vi "LabVIEWRTControlStartupVI.vi"() -> ()   [LabVIEW 2014]
doc: "This example demonstrates a command based communication architecture using TCP. It shows a protocol for packaging and parsing data while minimizing network traffic. Refer to the National Instruments Web site at ni.com/info and enter the info code \"commtcp\" for more information about this command based communication architecture."
uses:
  Control 2.ctl
  ChannelCommand.ctl
  Control 1.ctl
  WaveType.ctl
  MoterEnable.ctl
  <userlib>/VMIC/VMIC 5565 Reflective Memory.llb/VMIC Reference.ctl
  <vilib>/Platform/TimedLoop/XDataNode/timing_clust.ctl
  <vilib>/Platform/TimedLoop/XDataNode/nitl_modes.ctl
  <vilib>/Platform/TimedLoop/XDataNode/wakeup.ctl
  <vilib>/DAQmx/write.llb/DAQmx Write (Analog 1D DBL NChan 1Samp).vi
  <userlib>/VMIC/VMIC 5565 Reflective Memory.llb/VMIC Write (U32).vi
  <vilib>/DAQmx/write.llb/DAQmx Write (Digital 1D Bool NChan 1Samp 1Line).vi
  <userlib>/VMIC/VMIC 5565 Reflective Memory.llb/VMIC Read (U8).vi
  <vilib>/Platform/TimedLoop/XDataNode/XDataNode.xnode
  <vilib>/Platform/TimedLoop/XDataNode/XDNodeRunTimeDep.lvlib
  <vilib>/real-time/NI_Real-Time Libraries.lvlib
  <vilib>/NI_Real-Time Target Support.lvlib
  <vilib>/real-time/rtutility.llb/RT Restart Target (Self).vi
panel:
  out "Protect":bool
  out "x = y?":bool
  out "error out 12":errorcluster caption="错误输出"
  out "number of samples written per channel":u32
  out "error out 11":errorcluster caption="error out"
  out "error out 10":errorcluster caption="error out"
  out "error out 9":errorcluster caption="error out"
  out "上传数组":dbl[](array[numeric])
  out "VMIC write":sgl[](array[numeric])
  out "6612counterTask 8":refnum<k21>
  out "6612counterTask 7":refnum<k21>
  out "6612counterTask 6":refnum<k21>
  out "6612counterTask 5":refnum<k21>
  out "ResetAforce":dbl[](array[numeric])
  out "x/y":dbl
  out "全局结束时间":i64
  out "实际结束[i-1]":i64
  out "延迟完成？[i-1]":bool
  out "超时":i32=-1
  out "6612counterTask 4":refnum<k21>
  out "6612counterTask 3":refnum<k21>
  out "6612counterTask 2":refnum<k21> caption="任务输出"
  out "6612counterTask":refnum<k21>
  out "x与y? 4":bool[](array[boolean])
  out "x与y? 3":bool[](array[boolean])
  out "VMIC reference":T1
  out "PXI6363IO":refnum<k21>
  out "x与y?":bool[](array[boolean])
  out "error out 6":errorcluster caption="error out"
  out "error out 4":errorcluster
  out "OutPut":dbl[](array[numeric])
  out "Command Type":i32
  out "Msg Head":string
  out "error out":errorcluster caption="错误输出"
  out "长度 3":i32
  out "长度 2":i32
  out "长度":i32
  out "connection ID":refnum<k5> caption="连接ID"
  out "6363Task":refnum<k21> caption="任务输出"
  out "error out 3":errorcluster caption="错误输出"
  out "加速度信号":dbl[](array[numeric])
  out "同步信号":dbl[](array[numeric])
  out "轴向位移":dbl[](array[numeric])
  out "轴向力":dbl[](array[numeric])
  out "T_outrange":bool[](array[boolean])
  out "error out 8":errorcluster caption="error out"
  out "error out 7":errorcluster caption="error out"
  out "error out 5":errorcluster caption="错误输出"
  out "diff syn out 2":dbl[](array[numeric])
  out "Forward":dbl[](array[numeric])
  out "AngleSampleData 2":dbl[](array[numeric])
  out "TorqueSampledata 2":dbl[](array[numeric])
  out "control out":dbl[](array[numeric])
  out "command out 2":dbl[](array[numeric])
  out "Wave out 2":dbl[](array[numeric])
  out "type out":dbl[](array[numeric])
  out "Enable":bool[](array[boolean])
  out "syn out":dbl[](array[numeric])
  out "TempAnOut":dbl[](array[numeric])
  out "StartChannelReset":bool[](array[boolean])
  out "retorquedata2":dbl[](array[numeric])
  out "reangeldata2":dbl[](array[numeric])
  out "output 4":dbl[](array[numeric])
  out "TestLoops 2":i32
  out "ResetAngle":dbl[](array[numeric])
  out "ResetTorque":dbl[](array[numeric])
  out "error out 2":errorcluster
  in  "Exit":bool
  out "ControlPara":dbl[][](array[numeric])
  out "ChannelSetArray":T2 {"Enable" items=["不使能", "使能"]; "Wave" items=["0指令", "正弦波", "方波", "三角波", "常值", "波形数据", "白噪声", "正弦扫频", "梯度加载", "VMIC"]; "ChannelType" items=["标准波形跟踪"=1, "扫频测试"=2, "消除多余力"=3, "梯度加载"=4, "载荷谱跟踪"=5, "模拟输入跟踪"=9]; "ChannelStatus" items=["通道关", "位置通道", "加载通道"]}
  out "Stop":bool
  out "iCommand":i32
  out "TestLoops":i32
  out "dt":dbl
  out "PXI6733Task":refnum<k21>
  out "Data array":dbl[][](array[numeric])
  out "error  out":errorcluster
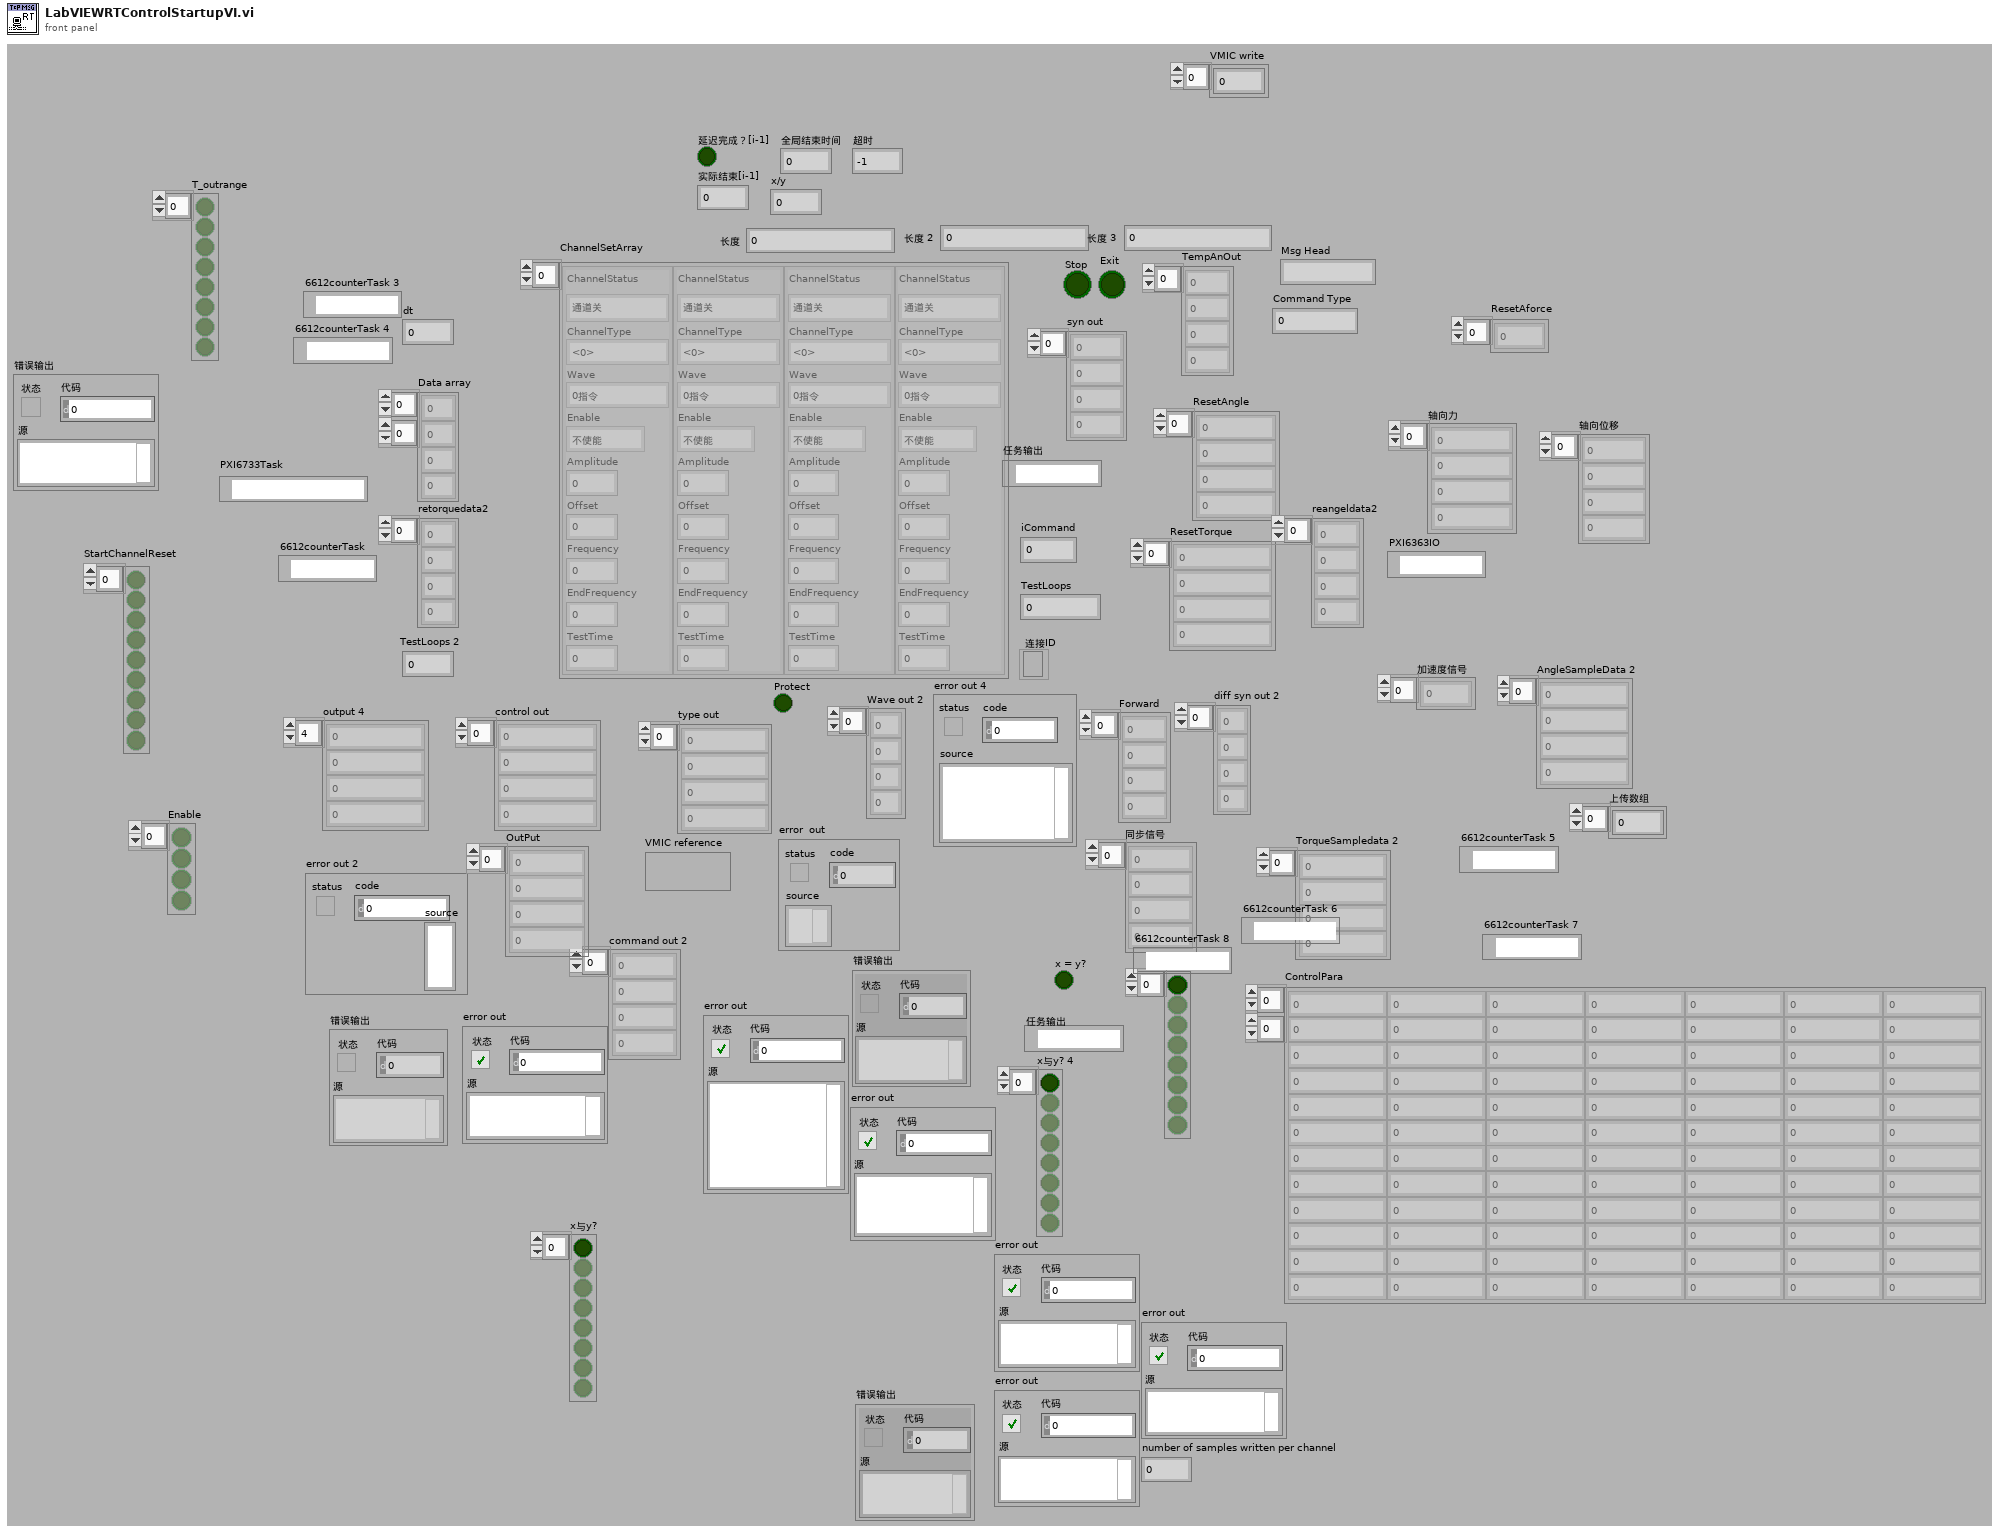
[diagram p1: front panel]
types:
  T1 = typedef "VMIC Reference.ctl" = variant
  T2 = typedef "Control 2.ctl" = T3[]
  T3 = typedef "ChannelCommand.ctl" = cluster{"ChannelStatus":T4, "ChannelType":i32, "Wave":T5, "Enable":T6, "Amplitude":dbl, "Offset":dbl, "Frequency":dbl, "EndFrequency":dbl, "TestTime":dbl}
  T4 = typedef "Control 1.ctl" = i32
  T5 = typedef "WaveType.ctl" = i32
  T6 = typedef "MoterEnable.ctl" = u16
  T7 = typedef "XDNodeRunTimeDep.lvlib/timing_clust.ctl" = cluster{"Expected End [f-1]":u64, "Actual End [f-1]":u64, "Finished Late? [f-1]":bool, "Expected End [i-1]":u64, "Actual End [i-1]":u64, "Finished Late? [i-1]":bool, "Expected Start [i]":u64, "Actual Start [i]":u64, "Expected Start [f]":u64, "Actual Start [f]":u64, "Source Name":string, "Structure Name":string, "Period":i64, "Deadline":i64, "Offset":i64, "Start":i64, "Priority":i32, "Timeout":i32, "Mode":T8, "Wakeup Reason":T9, "Error":errorcluster, "Source Type":string, "Secondary Source Type":string, "Global End Time":u64, "Global Start Time":u64, "Frame Duration":u64, "Iteration Duration":u64, "Assigned CPU":i32, "I/O Scan Engine Mode":u32}
  T8 = typedef "XDNodeRunTimeDep.lvlib/nitl_modes.ctl" = enum32{"No Change", "Process missed periods, maintain original phase", "Discard missed periods, maintain original phase", "Process missed periods, ignore original phase", "Discard missed periods, ignore original phase"}
  T9 = typedef "XDNodeRunTimeDep.lvlib/wakeup.ctl" = enum32{"Normal", "Aborted", "Asynchronous wakeup", "Timing source error", "Timed loop error", "Timeout"}
  T10 = enum16{"big-endian, network order", "native, host order", "little-endian"}
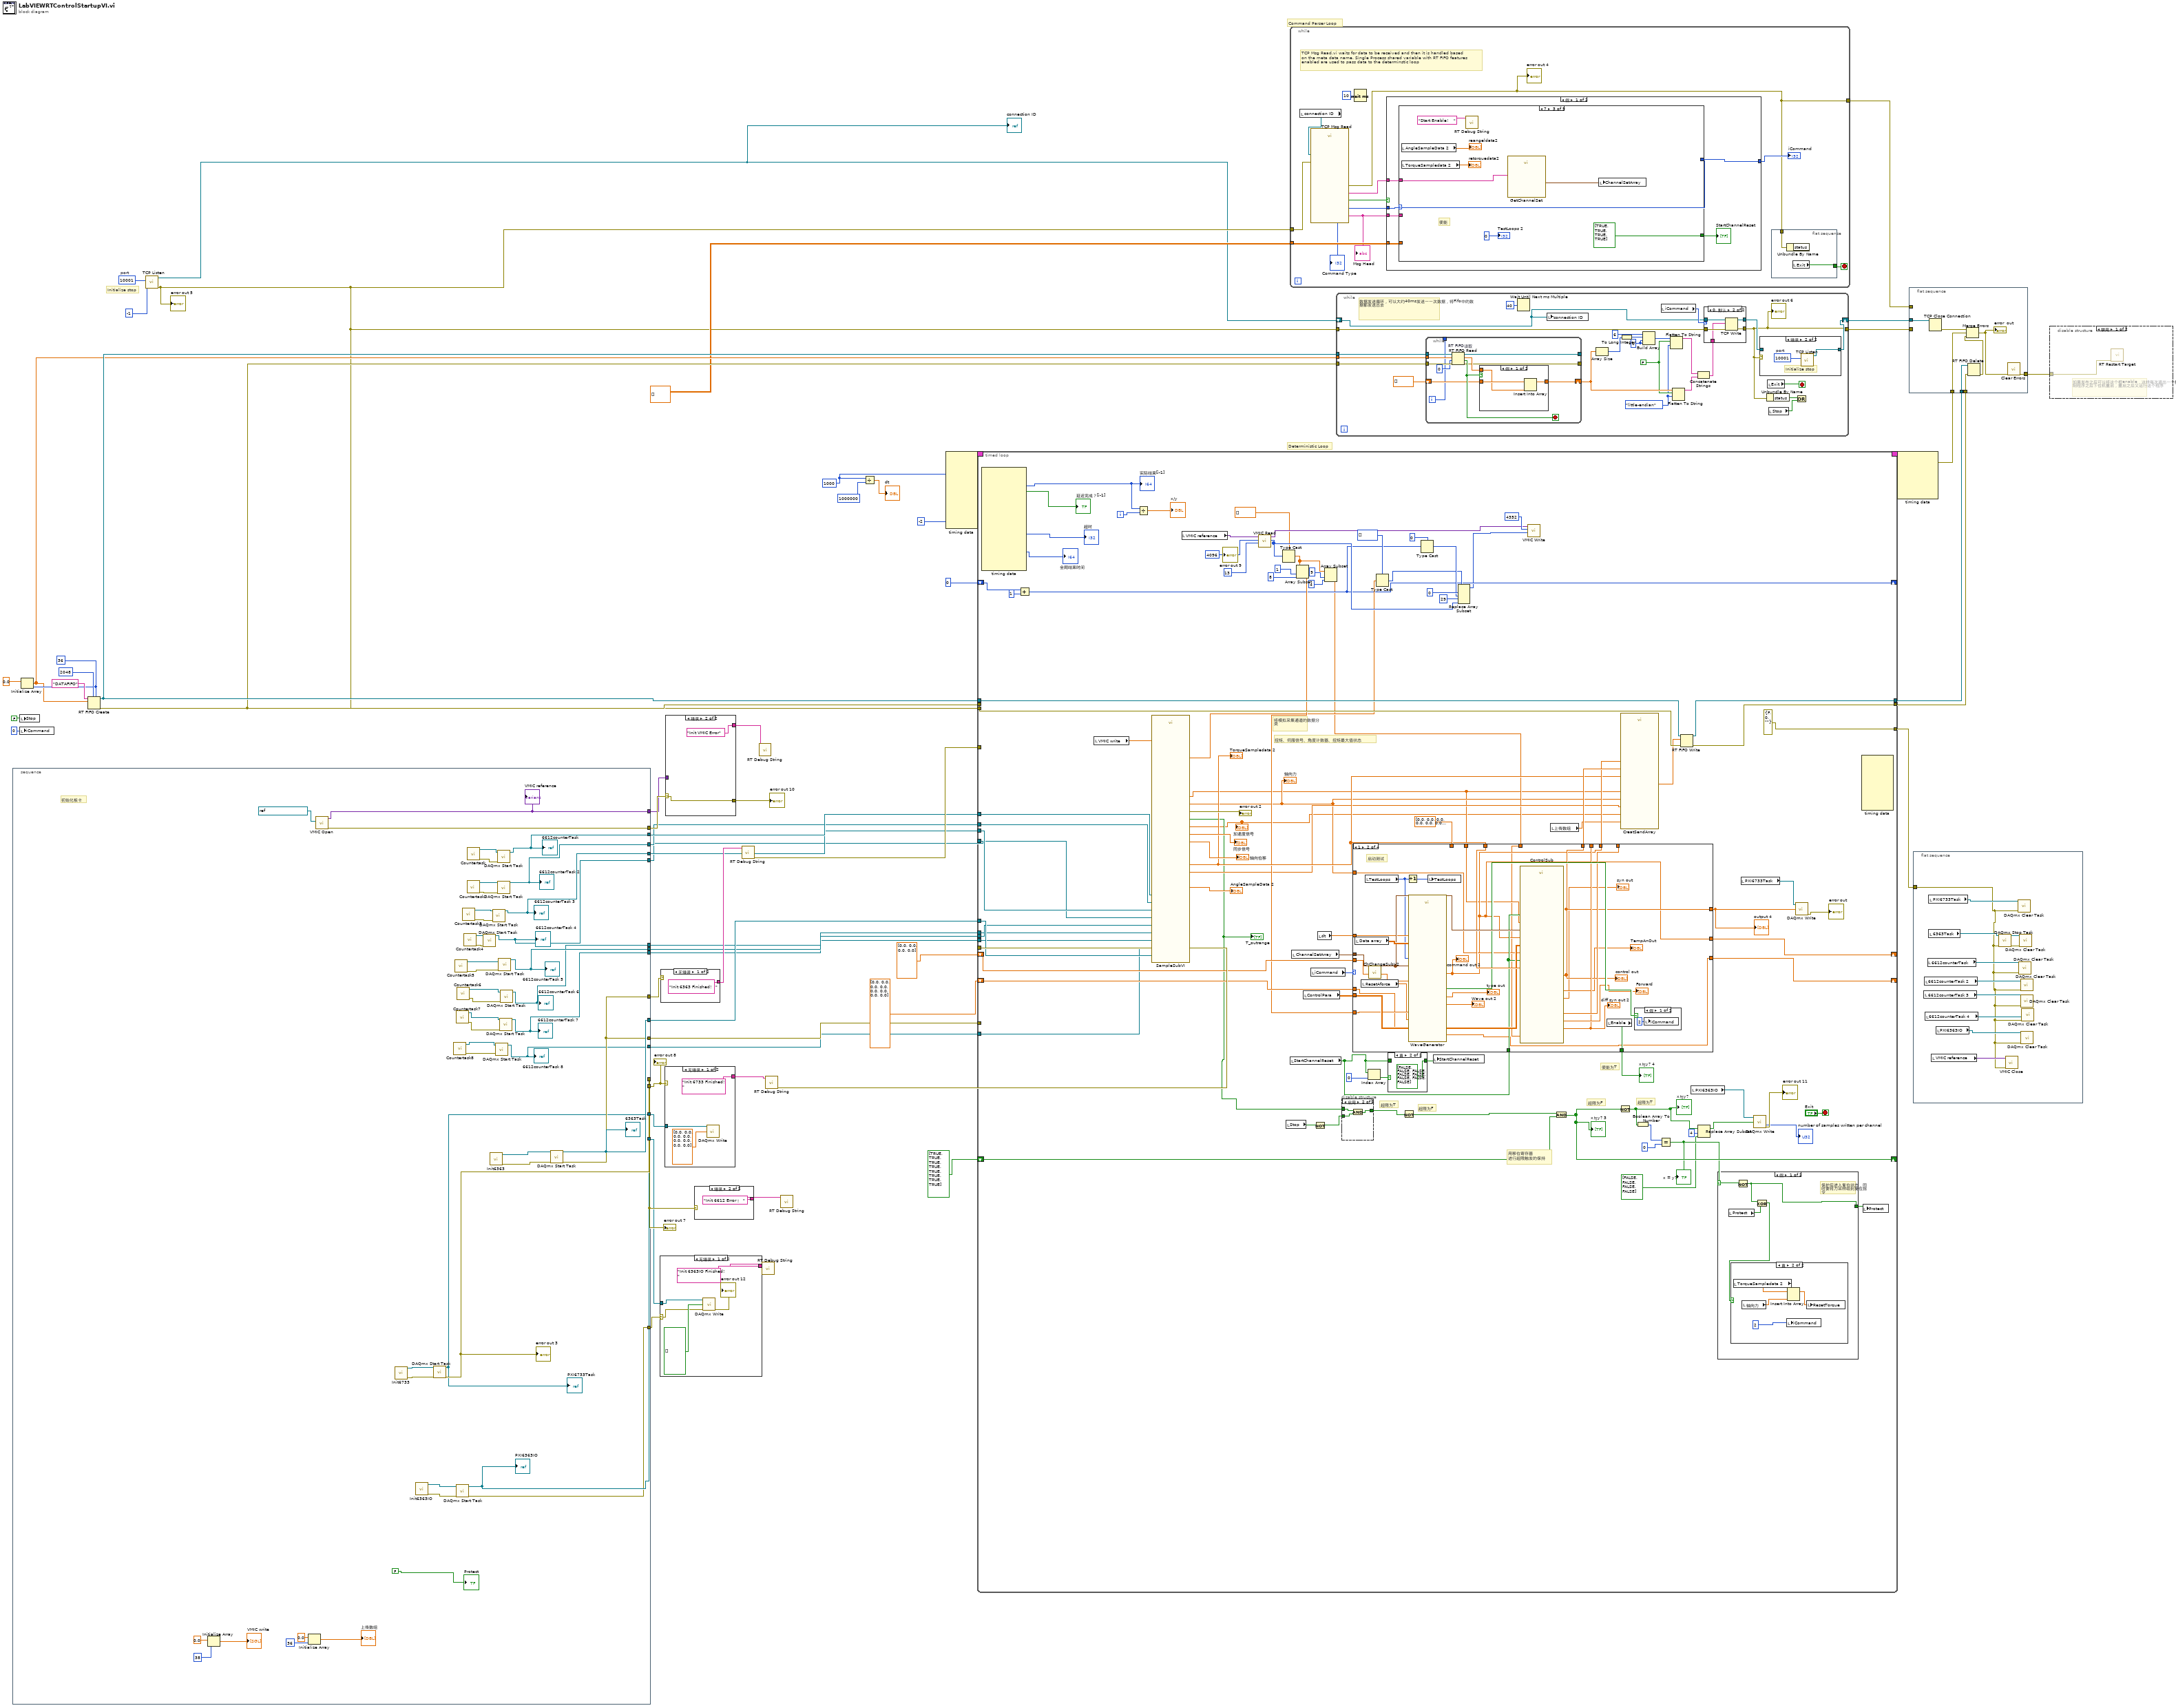
[diagram p0: block diagram]
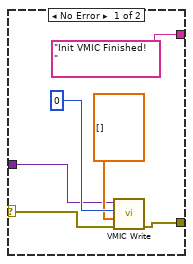
[diagram p2: hidden frame]
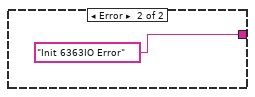
[diagram p3: hidden frame]
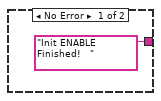
[diagram p4: hidden frame]
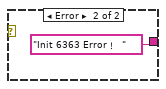
[diagram p5: hidden frame]
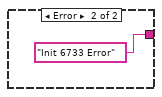
[diagram p7: hidden frame]
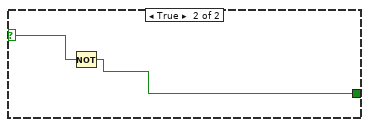
[diagram p9: hidden frame]
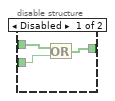
[diagram p10: hidden frame]
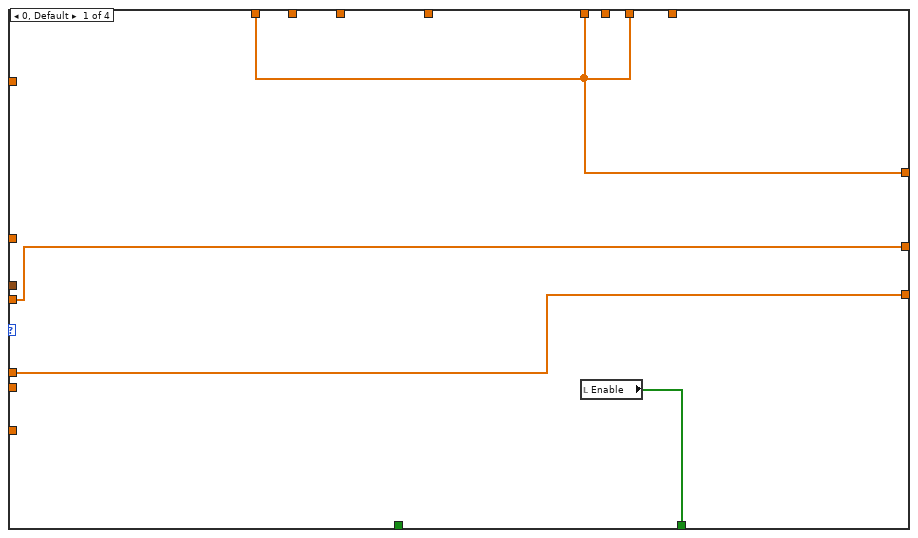
[diagram p12: hidden frame]
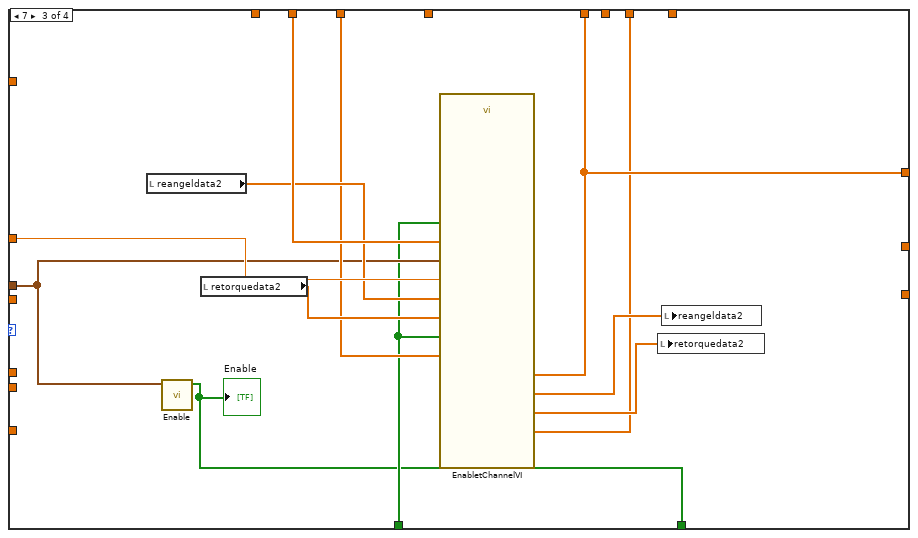
[diagram p14: hidden frame]
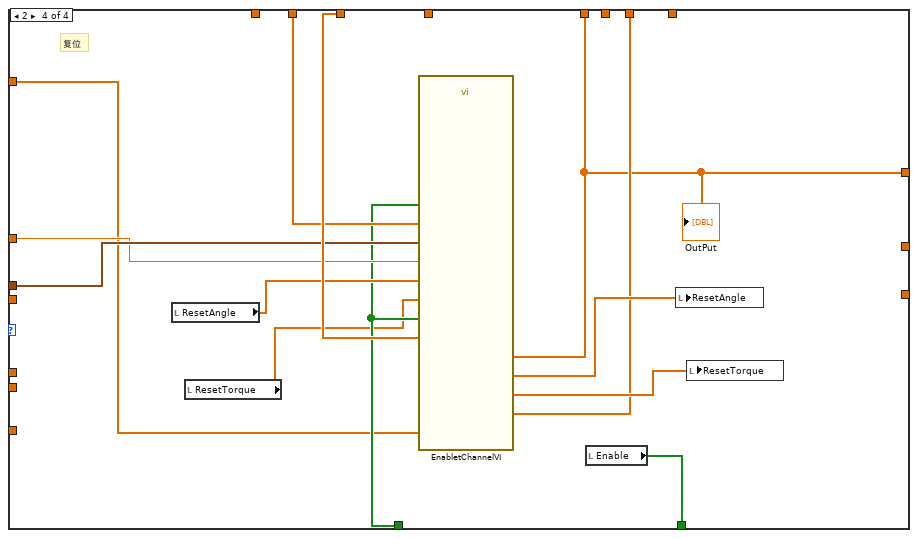
[diagram p15: hidden frame]
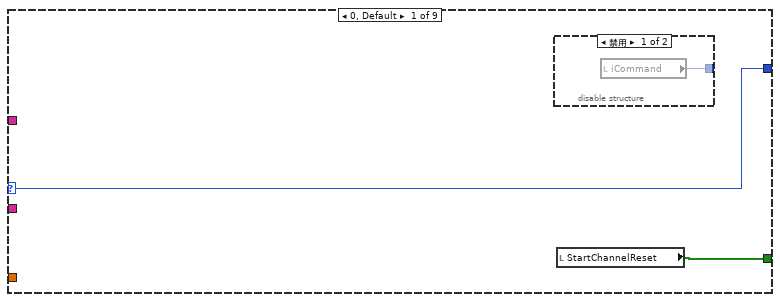
[diagram p16: hidden frame]
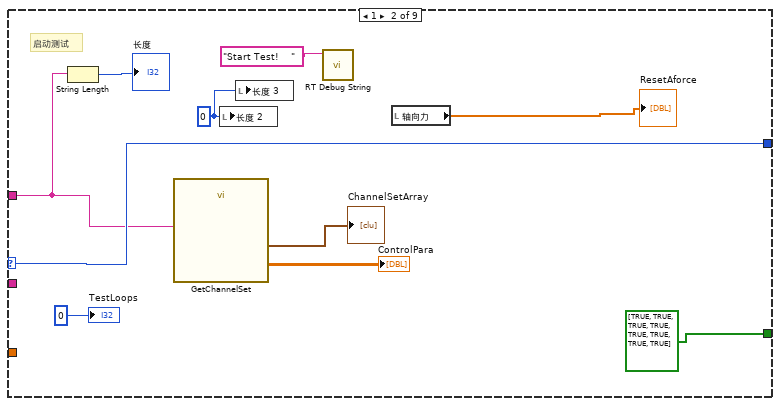
[diagram p18: hidden frame]
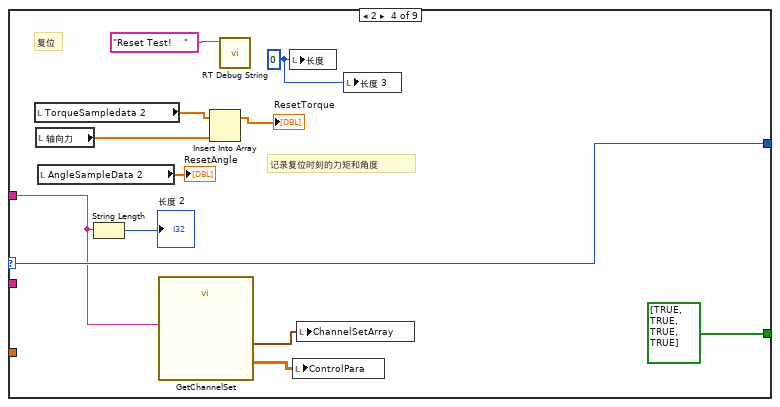
[diagram p19: hidden frame]
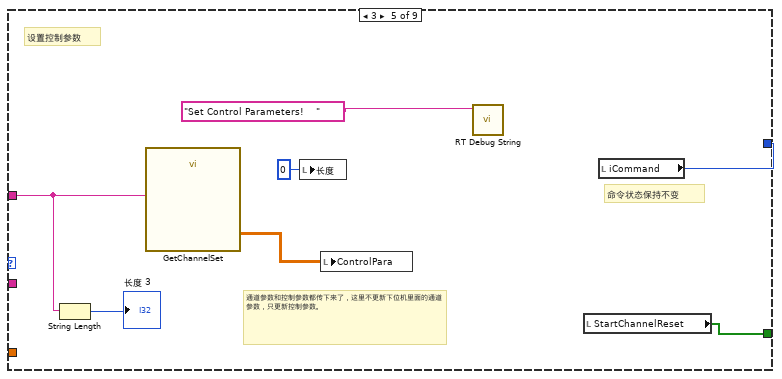
[diagram p20: hidden frame]
diagram:
  w46 = u32 36 ("elements in array (1)")
  w54 = i64 1000 ("Period")
  w58 = u16 10001  # port
  # "Deterministic Loop"
  # "Initialize stop"
  # "Command Parser Loop"
  n1 = stacked-sequence {
    tunnel: [w87] -> w25
    tunnel: [w87] -> w28
    tunnel: [w88] -> w24
    tunnel: [w85] -> w23
    tunnel: [w88] -> w9
    tunnel: [w89] -> w22
    tunnel: [w81] -> w17
    tunnel: [w83] -> w19
    tunnel: [w103] -> w16
    tunnel: [w102] -> w15
    tunnel: [w93] -> w13
    tunnel: [w92] -> w12
    tunnel: [w91] -> w11
    tunnel: [w90] -> w10
    tunnel: [w69] -> w8
    tunnel: [w68] -> w7
    tunnel: [w67] -> w6
    tunnel: [w66] -> w5
    frame #0 {
      # "初始化板卡"
      n2 = Initialize Array(sgl 0.0 ("元素"), 38 ("维数大小")) -> (→"VMIC write":sgl[])
      n3 = Initialize Array(0.0 ("element"), 36 ("dimension size")) -> (→"上传数组":dbl[])
      n4 = call <userlib>:"VMIC Open.vi"("VISA resource name (empty)"=refnum<visa-resource-name> "PXI13::12::INSTR") -> ("error out"=w103:errorcluster, "VMIC reference"=w102:T1)  [unwired: 5 in]
      "VMIC reference" <- w102
      n5 = call "Init6733.vi"() -> ("error out"=w84:errorcluster, "task out"=w86:refnum<k21>)  [unwired: 10 in]
      n6 = call "Init6363IO.vi"() -> ("error out"=w80:errorcluster, "task out"=w82:refnum<k21>)  [unwired: 10 in]
      n7 = call <vilib>:"DAQmx Start Task.vi"("task/channels in"=w86, "error in"=w84) -> ("task out"=w85:refnum<k21>, "error out"=w87:errorcluster)  [unwired: 12 in]
      "PXI6733Task" <- w85
      "error out 3" <- w87
      n8 = call "Countertask8.vi"() -> ("error out"=w70:errorcluster, "task out"=w71:refnum<k21>)  [unwired: 10 in]
      n9 = call "Countertask5.vi"() -> ("error out"=w76:errorcluster, "task out"=w77:refnum<k21>)  [unwired: 10 in]
      n10 = call "Countertask7.vi"() -> ("error out"=w72:errorcluster, "task out"=w73:refnum<k21>)  [unwired: 10 in]
      n11 = call <vilib>:"DAQmx Start Task.vi"("task/channels in"=w82, "error in"=w80) -> ("task out"=w83:refnum<k21>, "error out"=w81:errorcluster)  [unwired: 12 in]
      "PXI6363IO" <- w83
      n12 = call "Countertask6.vi"() -> ("error out"=w74:errorcluster, "task out"=w75:refnum<k21>)  [unwired: 10 in]
      n13 = call "Countertask3.vi"() -> ("error out"=w96:errorcluster, "task out"=w97:refnum<k21>)  [unwired: 10 in]
      n14 = call "Countertask4.vi"() -> ("error out"=w94:errorcluster, "task out"=w95:refnum<k21>)  [unwired: 10 in]
      n15 = call "Countertask2.vi"() -> ("error out"=w98:errorcluster, "task out"=w99:refnum<k21>)  [unwired: 10 in]
      n16 = call "Countertask.vi"() -> ("error out"=w100:errorcluster, "task out"=w101:refnum<k21>)  [unwired: 10 in]
      n17 = call <vilib>:"DAQmx Start Task.vi"("task/channels in"=w95, "error in"=w94) -> ("task out"=w90:refnum<k21>)  [unwired: 12 in, 1 out]
      "6612counterTask 4" <- w90
      n18 = call "Init6363.vi"() -> ("error out"=w78:errorcluster, "task out"=w79:refnum<k21>)  [unwired: 10 in]
      n19 = call <vilib>:"DAQmx Start Task.vi"("task/channels in"=w97, "error in"=w96) -> ("task out"=w91:refnum<k21>)  [unwired: 12 in, 1 out]
      "6612counterTask 3" <- w91
      n20 = call <vilib>:"DAQmx Start Task.vi"("task/channels in"=w71, "error in"=w70) -> ("task out"=w66:refnum<k21>)  [unwired: 12 in, 1 out]
      "6612counterTask 8" <- w66
      n21 = call <vilib>:"DAQmx Start Task.vi"("task/channels in"=w101, "error in"=w100) -> ("task out"=w93:refnum<k21>)  [unwired: 12 in, 1 out]
      "6612counterTask" <- w93
      n22 = call <vilib>:"DAQmx Start Task.vi"("task/channels in"=w99, "error in"=w98) -> ("task out"=w92:refnum<k21>)  [unwired: 12 in, 1 out]
      "6612counterTask 2" <- w92
      n23 = call <vilib>:"DAQmx Start Task.vi"("task/channels in"=w77, "error in"=w76) -> ("task out"=w69:refnum<k21>)  [unwired: 12 in, 1 out]
      "6612counterTask 5" <- w69
      n24 = call <vilib>:"DAQmx Start Task.vi"("task/channels in"=w73, "error in"=w72) -> ("task out"=w67:refnum<k21>)  [unwired: 12 in, 1 out]
      "6612counterTask 7" <- w67
      n25 = call <vilib>:"DAQmx Start Task.vi"("task/channels in"=w75, "error in"=w74) -> ("task out"=w68:refnum<k21>)  [unwired: 12 in, 1 out]
      "6612counterTask 6" <- w68
      n26 = call <vilib>:"DAQmx Start Task.vi"("task/channels in"=w79, "error in"=w78) -> ("task out"=w89:refnum<k21>, "error out"=w88:errorcluster)  [unwired: 12 in]
      "6363Task" <- w89
      "Protect" <- FALSE
    }
  }
  "error out 7" <- w28
  "error out 8" <- w25
  n27 = local write "Stop"(FALSE ("stop")) -> ()
  n28 = local write "iCommand"(0 ("iCommand")) -> ()
  n29 = Initialize Array(0.0, w46) -> (w45:dbl[])
  n30 = RT FIFO Create(0:"DATAFIFO" ("name (unnamed)"), 1:w45, 4:u32 2048 ("size (10)"), 6:w46) -> (8:w49:refnum<k33>, 11:w48:errorcluster)  [unwired: 4 in, 1 out]
  n31 = call <vilib>:"TCP Listen.vi"("timeout ms (wait forever: -1)"=-1, "port"=w58) -> ("error out"=w38:errorcluster, "connection ID"=w21:refnum<k5>)  [unwired: 2 in, 6 out]
  "error out 5" <- w38
  "connection ID" <- w21
  n32 = case shown="无错误" w17 {
    selector: w17 -> [w106 _]
    tunnel: ["Init 6363IO Finished!   " ("String to write") "Init 6363IO Error" ("String to write")] -> w18
    tunnel: w19 -> [w108 _]
    frame No Error {
      n33 = call-poly <vilib>:"DAQmx Write.vi"("task/channels in"=w108, "data"=bool[] [], "error in"=w106) -> ("error out"=→"error out 12":errorcluster)  [unwired: 10 in, 2 out]
    }
    frame Error {
    }
  }
  n34 = case shown="无错误" w24 {
    tunnel: ["Init 6363 Finished!   " ("String to write") "Init 6363 Error！  " ("String to write")] -> w37
    frame No Error {
    }
    frame Error {
    }
  }
  n35 = case shown="无错误" w25 {
    tunnel: ["Init 6733 Finished!   " ("String to write") "Init 6733 Error" ("String to write")] -> w34
    tunnel: w23 -> [w113 _]
    frame No Error {
      n36 = call-poly <vilib>:"DAQmx Write.vi"("task/channels in"=w113, "data"=dbl[] [0.0, 0.0, 0.0, 0.0, 0.0, 0.0, 0.0, 0.0]) -> ()  [unwired: 11 in, 3 out]
    }
    frame Error {
    }
  }
  n37 = case shown="错误" w16 {
    selector: w16 -> [w121 w123]
    tunnel: ["Init VMIC Finished!   " ("String to write") "Init VMIC Error" ("String to write")] -> w14
    tunnel: w15 -> [w118 _]
    tunnel: [w117 w123] -> w2
    frame No Error {
      n38 = call-poly <userlib>:"VMIC Write.vi"("error in (no error)"=w121, "buffer"=dbl[] [], "offset (0)"=u32 0, "VMIC reference in"=w118) -> ("error out"=w117:errorcluster)  [unwired: 2 in, 1 out]
    }
    frame Error {
    }
  }
  "error out 10" <- w2
  n39 = case shown="错误" w28 {
    tunnel: ["Init ENABLE Finished!   " ("String to write") "Init 6612 Error！  " ("String to write")] -> w29
    frame No Error {
    }
    frame Error {
    }
  }
  n40 = call <vilib>:"RT Debug String.vi"("String to write"=w37) -> ("error out"=w36:errorcluster)  [unwired: 10 in]
  n41 = call <vilib>:"RT Debug String.vi"("String to write"=w14) -> ()  [unwired: 10 in, 1 out]
  n42 = call <vilib>:"RT Debug String.vi"("String to write"=w18) -> ()  [unwired: 10 in, 1 out]
  n43 = call <vilib>:"RT Debug String.vi"("String to write"=w34) -> ("error out"=w35:errorcluster)  [unwired: 10 in]
  n44 = call <vilib>:"RT Debug String.vi"("String to write"=w29) -> ()  [unwired: 10 in, 1 out]
  n45 = Divide(x=w54, y=i64 1000000) -> (x/y=→"dt":dbl)
  n46 = node-c288(-2 ("Processor"), w54) -> (w57:T7)  [unwired: 7 in, 1 out]
  n47 = timed-loop "Timed Loop" {
    timing: w57 -> [_]
    timing-out: [_] -> w56
    tunnel: w49 -> [w221]
    tunnel: w48 -> [w219]
    tunnel: [w220] -> w30
    tunnel: [w218] -> w31
    tunnel: [errorcluster {"status"=FALSE, "code"=0, "source"=""} ("error in")] -> w39
    tunnel: w38 -> [_]
    tunnel: w36 -> [_]
    tunnel: w35 -> [_]
    shift-right: [w173] -> _
    shift-left: dbl[] [0.0, 0.0, 0.0, 0.0, 0.0, 0.0, 0.0, 0.0] -> [w202]
    shift-right: [w201] -> _
    shift-left: dbl[] [0.0, 0.0, 0.0, 0.0] -> [w200]
    tunnel: w22 -> [w197]
    tunnel: w9 -> [_]
    shift-right: [w140] -> _
    shift-left: bool[] [TRUE, TRUE, TRUE, TRUE, TRUE, TRUE, TRUE, TRUE] -> [w190]
    tunnel: w13 -> [w186]
    tunnel: w12 -> [w185]
    tunnel: w11 -> [w184]
    tunnel: w10 -> [w183]
    tunnel: w8 -> [w177]
    tunnel: w7 -> [w176]
    tunnel: w6 -> [w175]
    tunnel: w5 -> [w174]
    shift-right: [w158] -> _
    shift-left: 0 -> [w170]
    i -> [w179]
    stop <- "Exit" stop-if-true
    # "用移位寄存器\n进行超限触发的保持"
    # "使能为T"
    # "超限为T"
    # "超限为F"
    # "超限为T"
    # "超限为F"
    # "扭矩、伺服信号、角度计数器、扭矩最大值状态"
    # "将模拟采集通道的数据分类"
    n48 = node-c288() -> (w180:i64, →"延迟完成？[i-1]":bool, →"超时":i32, →"全局结束时间":i64)  [unwired: 13 out]
    "实际结束[i-1]" <- w180
    n49 = Add(x=w170, y=1) -> (x+y=w158:i32)
    n50 = local read "VMIC write"() -> (w157:sgl[])
    n51 = Divide(x=w180, y=w179) -> (x/y=→"x/y":dbl)
    n52 = call "SampleSubVI.vi"("task out"=w197, "Courter 1"=w186, "Courter 4"=w183, "Courter 2"=w185, "数组"=w157, "Courter 3"=w184, "Courter 7"=w175, "Courter 5"=w177, "Courter 8"=w174, "Courter 6"=w176) -> ("轴向位移"=→"轴向位移":dbl[], "轴向力"=w136:dbl[], "vmic反馈数据"=w159:sgl[], "AngleSample"=w162:dbl[], "加速度信号"=w128:dbl[], "同步信号"=→"同步信号":dbl[], "AngleSample 2"=→"AngleSampleData 2":dbl[], "F_outrange"=w131:bool[], "error out"=→"error out 2":errorcluster, "PositionSampleData"=w129:dbl[], "TorqueSample"=w172:dbl[])  [unwired: 3 in, 4 out]
    "TorqueSampledata 2" <- w172
    "T_outrange" <- w131
    "轴向力" <- w136
    "加速度信号" <- w128
    n53 = local read "VMIC reference"() -> (w151:T1)
    n54 = call-poly <userlib>:"VMIC Read.vi"("length (0)"=u32 13, "offset (0)"=u32 4096, "VMIC reference in"=w151) -> ("buffer"=w163:u32[], "VMIC reference out"=w155:T1)  [unwired: 2 in, 1 out]
    n55 = Type Cast(type=sgl[] [], x=w163) -> (*(type *) &x=w146:sgl[])
    n56 = local read "Stop"() -> (w193:bool)
    n57 = local read "StartChannelReset"() -> (w204:bool[])
    n58 = local read "ChannelSetArray"() -> (w212:T2)
    n59 = Array Subset(array=w146, index=1 ("索引"), length=8 ("长度")) -> (w168:sgl[])
    n60 = local read "ControlPara"() -> (w210:dbl[][])
    n61 = local read "iCommand"() -> (w209:i32)
    n62 = Not(x=w193) -> (.not. x?=w192:bool)
    n63 = local read "dt"() -> (w211:dbl)
    n64 = Array Subset(array=w146, index=9 ("索引"), length=4 ("长度")) -> (w143:sgl[])
    n65 = disable-structure shown="启用" {
      disable-tunnel: w192 -> [w239 w242]
      disable-tunnel: w131 -> [w238 w241]
      disable-tunnel: [w237 w240] -> w189
      frame Disabled {
        n66 = Or(x=w238, y=w239) -> (x .or. y?=w237:bool[])
      }
      frame Enabled {
        n67 = And(x=w241, y=w242) -> (x .and. y?=w240:bool[])
      }
    }
    n68 = case shown="1" w209 {
      tunnel: [w247 w255 w279 w294] -> w203
      tunnel: [w247 w256 w281 w292] -> w217
      tunnel: dbl[] [0.0, 0.0, 0.0, 0.0, 0.0, 0.0, 0.0, 0.0] ("Command") -> [w247 _ _ _]
      tunnel: [w247 w256 w281 w292] -> w208
      tunnel: w129 -> [_ w254 w289 w299]
      tunnel: w172 -> [_ w273 w285 w300]
      tunnel: w212 -> [_ w274 w284 w298]
      tunnel: w211 -> [_ w262 w288 w297]
      tunnel: w210 -> [_ w263 _ _]
      tunnel: w204 -> [_ w261 w280 w295]
      tunnel: [w248 w272 w278 w293] -> w187
      tunnel: w202 -> [w245 w250 _ _]
      tunnel: [w245 w249 _ _] -> w173
      tunnel: [_ w267 _ _] -> _
      tunnel: [_ w264 _ _] -> _
      tunnel: [w246 w255 _ _] -> w201
      tunnel: w200 -> [w246 w266 _ _]
      tunnel: w136 -> [_ w258 _ w291]
      tunnel: w168 -> [_ w260 _ _]
      tunnel: w143 -> [_ w251 _ _]
      frame 0, Default {
        n69 = local read "Enable"() -> (w248:bool[])
      }
      frame 1 {
        # "启动测试"
        n70 = local read "Data array"() -> (w275:dbl[][])
        n71 = local read "ResetAforce"() -> (w257:dbl[])
        n72 = local read "TestLoops"() -> (w259:i32)
        n73 = call "ChChangeSubV2.vi"("data in"=w266) -> ("data out"=w265:dbl[])  [unwired: 10 in]
        n74 = Increment(x=w259) -> (x+1=w276:i32)
        n75 = call "WaveGenerator.vi"("Data array"=w275, "dt"=w262, "TestLoops"=w259, "VMIC command"=w260, "WaveDefineArray"=w274, "Angle"=w265, "AxisForce"=w257, "LastVMICcommand"=w250) -> ("wave out 2"=→"Wave out 2":dbl[], "Command"=w255:dbl[], "Boolean"=w271:bool, "VMICafterFilter"=w249:dbl[], "type out"=→"type out":dbl[])  [unwired: 3 in]
        "command out 2" <- w255
        n76 = local write "TestLoops"(w276) -> ()
        n77 = call "ControlSub.vi"("AxisForceSample"=w258, "Command"=w255, "Angel"=w261, "AngleSample"=w254, "TorqueSample"=w273, "Torque"=w261, "syn-error"=w251, "ChannelSetArray"=w274, "ControlPara"=w263) -> ("syn out"=→"syn out":dbl[], "diff syn out 2"=w264:dbl[], "ControlOutput"=w256:dbl[], "Forward"=→"Forward":dbl[], "TempAnOut"=→"TempAnOut":dbl[], "control out"=w267:dbl[])  [unwired: 4 in, 1 out]
        "control out" <- w256
        "diff syn out 2" <- w264
        n78 = local read "Enable"() -> (w272:bool[])
        n79 = case shown="假" w271 {
          frame False {
            n80 = local write "iCommand"(2 ("iCommand")) -> ()
          }
          frame True {
          }
        }
      }
      frame 7 {
        n81 = local read "reangeldata2"() -> (w287:dbl[])
        n82 = call "Enable.vi"("ChannelSetArray2"=w284) -> ("Enable"=w278:bool[])  [unwired: 10 in]
        "Enable" <- w278
        n83 = local read "retorquedata2"() -> (w286:dbl[])
        n84 = call "EnabletChannelVI.vi"("Angelsample"=w289, "Angel"=w280, "dt"=w288, "Torquesample"=w285, "Torque"=w280, "ResetAngel"=w287, "ResetTorqueCommand"=w286, "ChannelSetArray"=w284) -> ("OutPut"=w281:dbl[], "resetAngel 2"=w282:dbl[], "ResetTorque 2"=w283:dbl[], "Commandout"=w279:dbl[])  [unwired: 4 in]
        n85 = local write "retorquedata2"(w283) -> ()
        n86 = local write "reangeldata2"(w282) -> ()
      }
      frame 2 {
        # "复位"
        n87 = local read "ResetAngle"() -> (w296:dbl[])
        n88 = local read "ResetTorque"() -> (w290:dbl[])
        n89 = call "EnabletChannelVI.vi"("Angelsample"=w299, "Angel"=w295, "dt"=w297, "Torquesample"=w300, "Torque"=w295, "ResetAngel"=w296, "ResetTorqueCommand"=w290, "ChannelSetArray"=w298, "AxisForceSample"=w291) -> ("OutPut"=w292:dbl[], "resetAngel 2"=w301:dbl[], "ResetTorque 2"=w302:dbl[], "Commandout"=w294:dbl[])  [unwired: 3 in]
        "OutPut" <- w292
        n90 = local read "Enable"() -> (w293:bool[])
        n91 = local write "ResetAngle"(w301) -> ()
        n92 = local write "ResetTorque"(w302) -> ()
      }
    }
    "output 4" <- w208
    "x与y? 4" <- w187
    n93 = Index Array(array=w204, index=0) -> (element=w207:bool)
    n94 = Type Cast(type=u32[] [], x=w159) -> (*(type *) &x=w161:u32[])
    n95 = case shown="真" w207 {
      tunnel: [w243 bool[] [FALSE, FALSE, FALSE, FALSE, FALSE, FALSE, FALSE, FALSE]] -> w205
      tunnel: w204 -> [w243 _]
      frame False {
      }
      frame True {
      }
    }
    n96 = Not(x=w189) -> (.not. x?=w188:bool[])
    n97 = Type Cast(type=u32 0, x=w158) -> (*(type *) &x=w165:u32)
    n98 = local write "StartChannelReset"(w205) -> ()
    n99 = Replace Array Subset(array=w161, new element #1=w165, index #1=0 ("索引"), new element #2=w163, index #2=29 ("索引")) -> (w154:u32[])
    n100 = call-poly <userlib>:"VMIC Write.vi"("buffer"=w154, "offset (0)"=u32 4352, "VMIC reference in"=w155) -> ()  [unwired: 3 in, 2 out]
    n101 = local read "上传数组"() -> (w127:dbl[])
    n102 = And(x=w188, y=w190) -> (x .and. y?=w140:bool[])
    "x与y? 3" <- w140
    n103 = Not(x=w140) -> (.not. x?=w135:bool[])
    "x与y?" <- w135
    n104 = call "CreatSendArray.vi"("AngleSample"=w162, "AxisForces"=w136, "AccumulateSample"=w128, "数组"=w127, "DisplacementSample"=w129, "ControlOutput"=w217, "TorqueSampledata"=w172, "Command"=w203) -> ("SendArray"=w216:dbl[])  [unwired: 3 in]
    n105 = Boolean Array To Number(Boolean array=w135) -> (number=w139:u32)
    n106 = Equal?(x=w139, y=u32 0) -> (x = y?=w137:bool)
    "x = y?" <- w137
    n107 = RT FIFO Write(0:w221, 1:w216, 3:w219) -> (8:w220:refnum<k33>, 11:w218:errorcluster)  [unwired: 2 in, 2 out]
    n108 = local read "PXI6363IO"() -> (w191:refnum<k21>)
    n109 = Replace Array Subset(array=w135, new element=bool[] [FALSE, FALSE, FALSE, FALSE], index=4 ("索引")) -> (w132:bool[])
    n110 = case shown="假" w137 {
      selector: w137 -> [w224 w231]
      tunnel: [w222 w230] -> w130
      frame False {
        # "保护后进入复位状态，同时要将力采样给到复位指令"
        n111 = local read "Protect"() -> (w225:bool)
        n112 = Not(x=w224) -> (.not. x?=w222:bool)
        n113 = Exclusive Or(1:w225, 2:w222) -> (0:w223:bool)
        n114 = case shown="真" w223 {
          frame False {
          }
          frame True {
            n115 = local read "TorqueSampledata 2"() -> (w228:dbl[])
            n116 = local read "轴向力"() -> (w229:dbl[])
            n117 = local write "iCommand"(2 ("iCommand")) -> ()
            n118 = Insert Into Array(array=w228, new element=w229) -> (w227:dbl[])  [unwired: 1 in]
            n119 = local write "ResetTorque"(w227) -> ()
          }
        }
      }
      frame True {
        n120 = Not(x=w231) -> (.not. x?=w230:bool)
      }
    }
    n121 = local read "PXI6733Task"() -> (w194:refnum<k21>)
    n122 = call-poly <vilib>:"DAQmx Write.vi"("task/channels in"=w191, "data"=w132) -> ("number of samples written per channel"=→"number of samples written per channel":u32, "error out"=→"error out 11":errorcluster)  [unwired: 11 in, 1 out]
    n123 = call-poly <vilib>:"DAQmx Write.vi"("task/channels in"=w194, "data"=w208) -> ("error out"=→"error out":errorcluster)  [unwired: 11 in, 2 out]
    n124 = node-c288() -> ()  [unwired: 7 in, 2 out]
    n125 = local write "Protect"(w130) -> ()
  }
  n126 = while {
    tunnel: w38 -> [w314]
    tunnel: [w307] -> w32
    tunnel: dbl[][] [] -> [w311]
    stop <- w306 stop-if-true
    # "TCP Msg Read.vi waits for data to be received and then it is handled based \non the meta data name. Single Process shared variable with RT FIFO features \nenabled are used to pass data to the determinstic loop"
    n127 = local read "connection ID"() -> (w304:refnum<k5>)
    n128 = call "TCP Msg Read.vi"("connection ID"=w304, "error in"=w314) -> ("Timed Out?"=w313:bool, "Command Type"=w309:i32, "Msg Data"=w312:string, "Msg Head"=w310:string, "error out"=w307:errorcluster)  [unwired: 12 in, 1 out]
    "Msg Head" <- w310
    "Command Type" <- w309
    "error out 4" <- w307
    n129 = Wait (ms)(milliseconds to wait=u32 10 ("等待时间（毫秒）")) -> ()  [unwired: 1 out]
    n130 = case shown="假" w313 {
      tunnel: w312 -> [w322 _]
      tunnel: w309 -> [w321 _]
      tunnel: w311 -> [w320 _]
      tunnel: w310 -> [w319 _]
      tunnel: [w318 w380] -> w308
      frame False {
        n131 = case shown="7" w321 {
          selector: w321 -> [w324 w331 w340 w353 _ w364 w374 w376 _]
          tunnel: w322 -> [_ w329 w343 w347 w357 w371 _ _ _]
          tunnel: w320 -> [_ _ _ _ _ w370 _ _ _]
          tunnel: w319 -> [_ _ _ _ _ w365 _ _ _]
          tunnel: [w324 w331 w340 w353 w360 w364 w374 w376 w379] -> w318
          tunnel: [w323 bool[] [TRUE, TRUE, TRUE, TRUE, TRUE, TRUE, TRUE, TRUE] bool[] [TRUE, TRUE, TRUE, TRUE] bool[] [TRUE, TRUE, TRUE, TRUE] w359 w363 w373 w375 w378] -> w317
          frame 0, Default {
            n132 = disable-structure shown="禁用" {
              disable-tunnel: [w325 _] -> _
              frame Disabled {
                n133 = local read "iCommand"() -> (w325:i32)
              }
              frame Enabled {
              }
            }
            n134 = local read "StartChannelReset"() -> (w323:bool[])
          }
          frame 1 {
            w327 = 0 ("长度 2")
            # "启动测试"
            n135 = String Length(string=w329) -> (length=→"长度":i32)
            n136 = call "GetChannelSet.vi"("Msg Data"=w329) -> ("ControlPara"=→"ControlPara":dbl[][], "ChannelSetArray"=→"ChannelSetArray":T3[])  [unwired: 9 in]
            n137 = local write "长度 2"(w327) -> ()
            n138 = local write "长度 3"(w327) -> ()
            n139 = call <vilib>:"RT Debug String.vi"("String to write"="Start Test!    ") -> ()  [unwired: 10 in, 1 out]
            n140 = local read "轴向力"() -> (→"ResetAforce":dbl[])
            "TestLoops" <- 0 ("TestLoops")
          }
          frame 7 {
            # "使能"
            n141 = local read "AngleSampleData 2"() -> (→"reangeldata2":dbl[])
            n142 = local read "TorqueSampledata 2"() -> (→"retorquedata2":dbl[])
            n143 = call <vilib>:"RT Debug String.vi"("String to write"="Start Enable!    ") -> ()  [unwired: 10 in, 1 out]
            n144 = call "GetChannelSet.vi"("Msg Data"=w343) -> ("ChannelSetArray"=w337:T3[])  [unwired: 9 in, 1 out]
            n145 = local write "ChannelSetArray"(w337) -> ()
            "TestLoops 2" <- 0 ("TestLoops")
          }
          frame 2 {
            w344 = 0 ("长度")
            # "记录复位时刻的力矩和角度"
            # "复位"
            n146 = local read "TorqueSampledata 2"() -> (w350:dbl[])
            n147 = local read "轴向力"() -> (w349:dbl[])
            n148 = local read "AngleSampleData 2"() -> (→"ResetAngle":dbl[])
            n149 = String Length(string=w347) -> (length=→"长度 2":i32)
            n150 = call "GetChannelSet.vi"("Msg Data"=w347) -> ("ControlPara"=w345:dbl[][], "ChannelSetArray"=w346:T3[])  [unwired: 9 in]
            n151 = Insert Into Array(array=w350, new element=w349) -> (→"ResetTorque":dbl[])  [unwired: 1 in]
            n152 = call <vilib>:"RT Debug String.vi"("String to write"="Reset Test!    ") -> ()  [unwired: 10 in, 1 out]
            n153 = local write "长度"(w344) -> ()
            n154 = local write "ControlPara"(w345) -> ()
            n155 = local write "ChannelSetArray"(w346) -> ()
            n156 = local write "长度 3"(w344) -> ()
          }
          frame 3 {
            # "命令状态保持不变"
            # "通道参数和控制参数都传下来了，这里不更新下位机里面的通道参数，只更新控制参数。"
            # "设置控制参数"
            n157 = String Length(string=w357) -> (length=→"长度 3":i32)
            n158 = call "GetChannelSet.vi"("Msg Data"=w357) -> ("ControlPara"=w362:dbl[][])  [unwired: 9 in, 1 out]
            n159 = local write "长度"(0 ("长度")) -> ()
            n160 = local write "ControlPara"(w362) -> ()
            n161 = call <vilib>:"RT Debug String.vi"("String to write"="Set Control Parameters!    ") -> ()  [unwired: 10 in, 1 out]
            n162 = local read "StartChannelReset"() -> (w359:bool[])
            n163 = local read "iCommand"() -> (w360:i32)
          }
          frame 6 {
            # "波形数据"
            n164 = call "TCP Data Read.vi"("Data"=w371, "Head"=w365) -> ("Data Channel"=w366:i32, "DataArray"=w369:dbl[])  [unwired: 8 in]
            n165 = Replace Array Subset(array=w370, new element=w369, index (row)=w366) -> (→"Data array":dbl[][])  [unwired: 1 in]
            n166 = local read "StartChannelReset"() -> (w363:bool[])
            n167 = disable-structure shown="Disabled" {
              disable-tunnel: [w372 _] -> _
              frame Disabled {
                n168 = local read "iCommand"() -> (w372:i32)
              }
              frame Enabled {
              }
            }
            n169 = call <vilib>:"RT Debug String.vi"("String to write"="Receive Wave Data\\n") -> ()  [unwired: 10 in, 1 out]
          }
          frame 4 {
            # "停止测试"
            n170 = local read "StartChannelReset"() -> (w373:bool[])
          }
          frame -1 {
            # "退出测试"
            n171 = local read "StartChannelReset"() -> (w375:bool[])
            "Stop" <- TRUE
          }
          frame 88 {
            # "看门狗指令"
            n172 = local read "StartChannelReset"() -> (w378:bool[])
            n173 = local read "iCommand"() -> (w379:i32)
          }
        }
        "StartChannelReset" <- w317
      }
      frame True {
        n174 = local read "iCommand"() -> (w380:i32)
      }
    }
    "iCommand" <- w308
    n175 = flat-sequence {
      tunnel: w307 -> [w316]
      tunnel: [w315] -> w306
      frame #0 {
        n176 = Unbundle By Name(w316) -> ()  [unwired: 1 out]
        n177 = local read "Exit"() -> (w315:bool)
      }
    }
  }
  n178 = while {
    tunnel: w38 -> [w403]
    tunnel: [w381] -> w33
    tunnel: w49 -> [w401]
    tunnel: w48 -> [w402]
    tunnel: w45 -> [w400]
    shift-right: [w383] -> w40
    shift-left: w21 -> [w382]
    stop <- w385 stop-if-true
    w388 = 0 ("element")
    w392 = FALSE ("prepend array or string size? (T)")
    w391 = T10."little-endian" ("byte order (0:big-endian, network order)")
    # "数据发送循环，可以大约40ms发送一一次数据，将Fifo中的数据都发送出去"
    n179 = while {
      tunnel: w401 -> [w426]
      tunnel: w402 -> [w425]
      tunnel: w400 -> [w424]
      shift-right: [w417] -> w396
      shift-left: dbl[] [] -> [w418]
      tunnel: [w422] -> _
      tunnel: [w419] -> _
      tunnel: [w416] -> _
      i -> [w416]
      stop <- w421 stop-if-true
      n180 = RT FIFO Read "RT FIFO读取"(0:w426, 1:w424, 2:0 ("timeout in ms (0)"), 3:w425) -> (8:w422:refnum<k33>, 9:w420:dbl[], 10:w421:bool, 11:w419:errorcluster)  [unwired: 1 out]
      n181 = case shown="假" w421 {
        tunnel: w420 -> [w427 _]
        tunnel: w418 -> [w429 w430]
        tunnel: [w428 w430] -> w417
        frame False {
          n182 = Insert Into Array(array=w429, new element=w427) -> (w428:dbl[])  [unwired: 1 in]
        }
        frame True {
        }
      }
    }
    n183 = Wait Until Next ms Multiple(millisecond multiple=u32 40) -> ()  [unwired: 1 out]
    n184 = local write "connection ID"(w382) -> ()
    n185 = Array Size(array=w396) -> (size(s)=w387:i32)
    n186 = To Long Integer(number=w387) -> (32bit integer=w389:i32)
    n187 = Build Array(6 ("data"), w389, w388, w388) -> (w393:i32[])
    n188 = local read "iCommand"() -> (w386:i32)
    n189 = Flatten To String(anything=w393, prepend array or string size? (T)=w392, byte order (0:big-endian, network order)=w391) -> (data string=w390:string)  [unwired: 1 in, 2 out]
    n190 = Flatten To String(anything=w396, prepend array or string size? (T)=w392, byte order (0:big-endian, network order)=w391) -> (data string=w395:string)  [unwired: 1 in, 2 out]
    n191 = Concatenate Strings(w390, w395) -> (w397:string)
    n192 = case shown="0, 默认" w386 {
      tunnel: w382 -> [w410 w415]
      tunnel: [w410 w414] -> w384
      tunnel: [w409 w413] -> w381
      tunnel: w403 -> [w409 w412]
      tunnel: w397 -> [_ w411]
      frame -1 {
      }
      frame 0, Default {
        n193 = TCP Write(connection ID=w415, data in=w411, error in (no error)=w412) -> (connection ID out=w414:refnum<k5>, error out=w413:errorcluster)  [unwired: 1 in, 1 out]
      }
    }
    "error out 6" <- w381
    n194 = case shown="错误" w381 {
      tunnel: w384 -> [w406 _]
      tunnel: [w406 w407] -> w383
      frame No Error {
      }
      frame Error {
        w408 = u16 10001  # port
        # "Initialize stop"
        n195 = call <vilib>:"TCP Listen.vi"("port"=w408) -> ("connection ID"=w407:refnum<k5>)  [unwired: 3 in, 7 out]
      }
    }
    n196 = Unbundle By Name(w381) -> ("status"=w404:bool)
    n197 = local read "Exit"() -> (w385:bool)
    n198 = local read "Stop"() -> (w399:bool)
    n199 = Or(x=w404, y=w399) -> ()  [unwired: 1 out]
  }
  n200 = node-c288(w56) -> (w55:errorcluster)  [unwired: 5 out]
  n201 = flat-sequence {
    tunnel: w55 -> [w438]
    tunnel: [w437] -> w27
    tunnel: w40 -> [w436]
    tunnel: w33 -> [_]
    tunnel: w32 -> [_]
    tunnel: w31 -> [w433]
    tunnel: w30 -> [w432]
    frame #0 {
      n202 = TCP Close Connection(connection ID=w436) -> (error out=w435:errorcluster)  [unwired: 1 in, 2 out]
      n203 = RT FIFO Delete(0:w432, 3:w433) -> (11:w431:errorcluster)  [unwired: 1 in]
      n204 = Merge Errors(w435, w438, w431) -> (w434:errorcluster)
      "error  out" <- w434
      n205 = call <vilib>:"Clear Errors.vi"("error in (no error)"=w434) -> ("error out"=w437:errorcluster)  [unwired: 5 in, 1 out]
    }
  }
  n206 = flat-sequence {
    tunnel: w39 -> [w439]
    frame #0 {
      n207 = local read "6612counterTask 3"() -> (w443:refnum<k21>)
      n208 = local read "6612counterTask 2"() -> (w444:refnum<k21>)
      n209 = local read "6612counterTask 4"() -> (w442:refnum<k21>)
      n210 = local read "6612counterTask"() -> (w445:refnum<k21>)
      n211 = local read "PXI6733Task"() -> (w446:refnum<k21>)
      n212 = local read "6363Task"() -> (w447:refnum<k21>)
      n213 = local read "VMIC reference"() -> (w440:T1)
      n214 = local read "PXI6363IO"() -> (w441:refnum<k21>)
      n215 = call <vilib>:"DAQmx Stop Task.vi"("task/channels in"=w447, "error in"=w439) -> ("task out"=w449:refnum<k21>, "error out"=w448:errorcluster)  [unwired: 12 in]
      n216 = call <userlib>:"VMIC Close.vi"("error in (no error)"=w439, "VMIC reference in"=w440) -> ()  [unwired: 5 in, 1 out]
      n217 = call <vilib>:"DAQmx Clear Task.vi"("task in"=w446, "error in"=w439) -> ()  [unwired: 13 in, 1 out]
      n218 = call <vilib>:"DAQmx Clear Task.vi"("task in"=w445, "error in"=w439) -> ()  [unwired: 13 in, 1 out]
      n219 = call <vilib>:"DAQmx Clear Task.vi"("task in"=w449, "error in"=w448) -> ()  [unwired: 13 in, 1 out]
      n220 = call <vilib>:"DAQmx Clear Task.vi"("task in"=w444, "error in"=w439) -> ()  [unwired: 13 in, 1 out]
      n221 = call <vilib>:"DAQmx Clear Task.vi"("task in"=w443, "error in"=w439) -> ()  [unwired: 13 in, 1 out]
      n222 = call <vilib>:"DAQmx Clear Task.vi"("task in"=w441, "error in"=w439) -> ()  [unwired: 13 in, 1 out]
      n223 = call <vilib>:"DAQmx Clear Task.vi"("task in"=w442, "error in"=w439) -> ()  [unwired: 13 in, 1 out]
    }
  }
  n224 = disable-structure shown="禁用" {
    disable-tunnel: w27 -> [w450 _]
    frame Disabled {
      # "如果发布之后可以将这个框enable，这样每次退出一个控制程序之后下位机重启，重启之后又运行这个程序"
      n225 = call-poly <vilib>:"RT Restart Target.vi"("error in (no error)"=w450) -> ()  [unwired: 10 in, 1 out]
    }
    frame Enabled {
    }
  }
